vi "Check Reference Type.vi"(8 "error in (no error)":errorcluster, 11 "Refnum Value Source in":refnum<class "Timestamp Ctrl Value Source.lvclass">) -> (0 "error out":errorcluster, 3 "Refnum Value Source out":refnum<class "Timestamp Ctrl Value Source.lvclass">)   [LabVIEW 2020, in "Composed Columns.lvlib" / "Timestamp Ctrl Value Source.lvclass"]
uses:
  Timestamp Ctrl Value Source.lvclass
  C:/Users/User/Desktop/Raman Program/Database OOP/source/Database OOP/Column Libraries/Ctrl Renum Value Source Class/Ctrl Refnum Value Source.lvclass
  Ctrl Renum Value Source Class/Ctrl Refnum Value Source.lvclass/Ctrl Refnum Value Source.ctl
  Ctrl Renum Value Source Class/Ctrl Refnum Value Source.lvclass
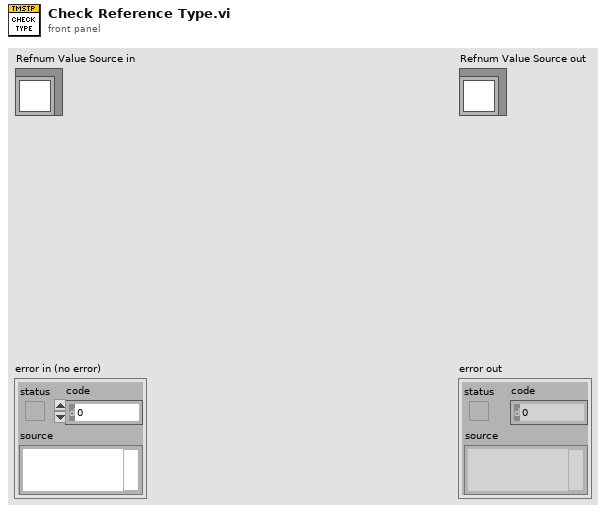
[diagram p1: front panel]
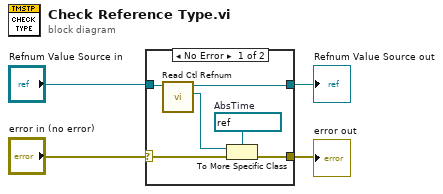
[diagram p0: block diagram]
diagram:
  n1 = case shown="No Error" "error in (no error)" {
    selector: "error in (no error)" -> [w5 w12]
    tunnel: [w9 w12] -> w2
    tunnel: "Refnum Value Source in" -> [w10 w11]
    tunnel: [w6 w11] -> w1
    frame No Error {
      w7 = refnum<vi> refnum  # AbsTime
      n2 = call "Read Ctl Refnum.vi"("Refnum Value Source in"=w10) -> ("Ctl Refnum"=w8:refnum<vi>, "Refnum Value Source out"=w6:refnum<class "Timestamp Ctrl Value Source.lvclass">)  [unwired: 8 in, 1 out]
      n3 = To More Specific Class(target class=w7, reference=w8, error in=w5) -> (error out=w9:errorcluster)  [unwired: 1 out]
    }
    frame Error {
    }
  }
  "error out" <- w2
  "Refnum Value Source out" <- w1
